vi "Manage Waypoint Shape.vi"(5 "Draw Arrow":bool, 6 "Coords":cluster{"x":dbl, "y":dbl}, 7 "Drawing Options":T1, 8 "Operation":enum16{"Draw", "Pt Test"}(ring), 9 "new picture in":picture, 10 "Waypoint Position (ft)":cluster{"x":dbl, "y":dbl, "th":dbl}, 11 "Pict Ref":refnum<vi>) -> (0 "Pt Test Results":enum16{"Miss", "Rect Hit", "Arrow Hit"}(ring), 1 "new picture out":picture)   [LabVIEW 2019]
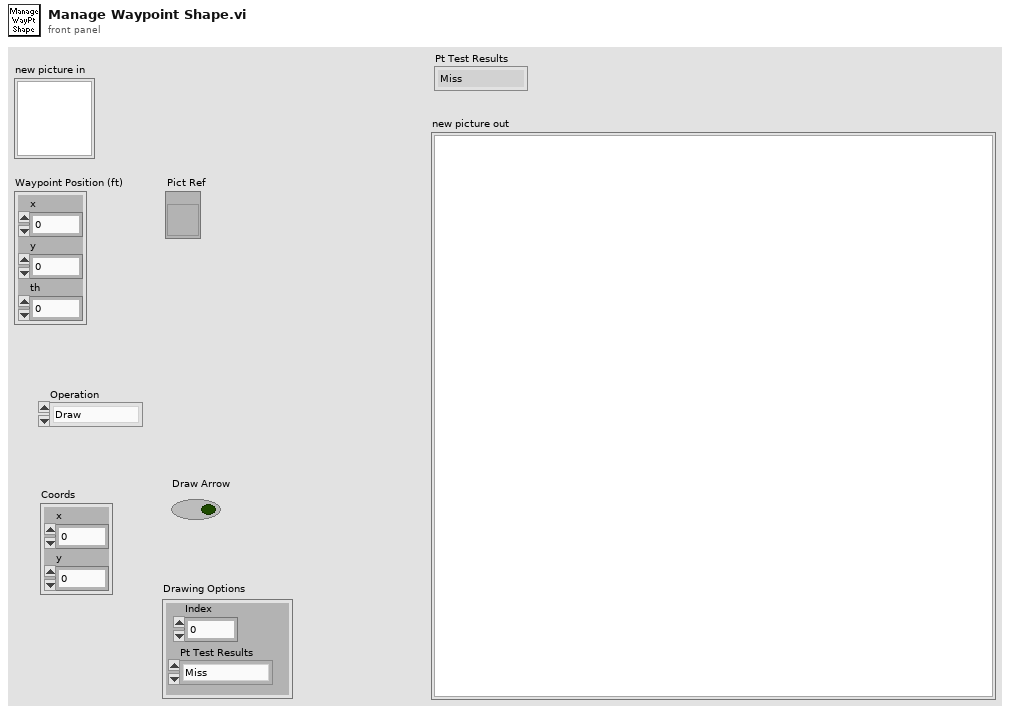
[diagram p1: front panel]
types:
  T1 = cluster{"Index":u32, "Pt Test Results":enum16{"Miss", "Rect Hit", "Arrow Hit"}}
  T2 = typedef "LVPositionTypeDef.ctl" = cluster{"Left":i32, "Top":i32}
  T3 = typedef "LVBoundsTypeDef.ctl" = cluster{"Width":u32, "Height":u32}
  T4 = cluster{"horizontal":enum16{"left", "center", "right"}, "vertical":enum16{"top", "center", "bottom"}}
  T5 = cluster{"Width":u16, "Style":enum32{"Solid", "Dash", "Dot", "DashDot", "DashDotDot"}}
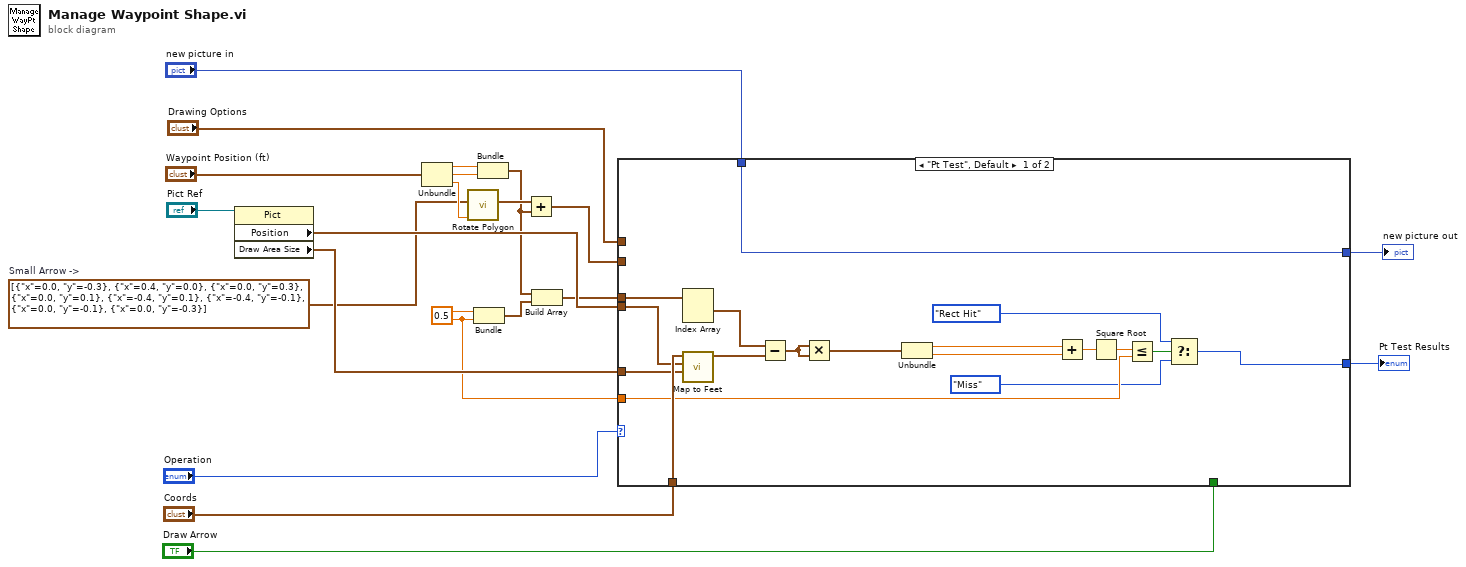
[diagram p0: block diagram]
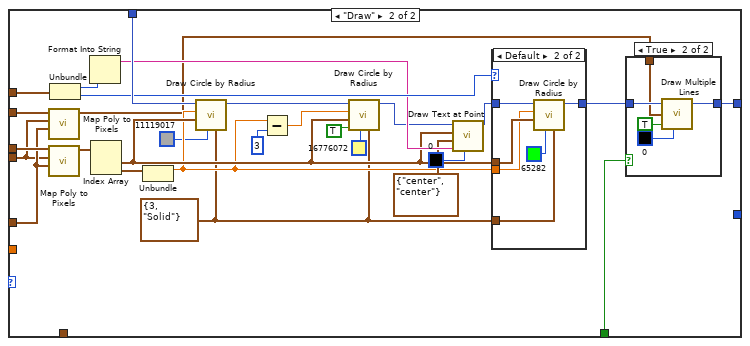
[diagram p2: hidden frame]
diagram:
  w5 = cluster{"x":dbl, "y":dbl}[] [{"x"=0.0, "y"=-0.3}, {"x"=0.4, "y"=0.0}, {"x"=0.0, "y"=0.3}, {"x"=0.0, "y"=0.1}, {"x"=-0.4, "y"=0.1}, {"x"=-0.4, "y"=-0.1}, {"x"=0.0, "y"=-0.1}, {"x"=0.0, "y"=-0.3}]  # Small Arrow ->
  w7 = 0.5 ("y")
  n1 = property on="Property Node" class="Pict"(reference="Pict Ref") -> ("Position"=w16:T2, "Draw Area Size"=w15:T3)  [unwired: 1 in, 2 out]
  n2 = Unbundle("Waypoint Position (ft)") -> ("x"=w18:dbl, "y"=w19:dbl, "th"=w6:dbl)
  n3 = call "Rotate Polygon.vi"("Angle"=w6, "polygon 2"=w5) -> ("polygon"=w4:cluster{dbl, dbl}[])  [unwired: 9 in]
  n4 = Bundle("y"=w7, "y"=w7) -> (w8:cluster{"y":dbl, "y":dbl})  [unwired: 1 in]
  n5 = Bundle("x"=w18, "y"=w19) -> (w3:cluster{"x":dbl, "y":dbl})  [unwired: 1 in]
  n6 = Add(x=w4, y=w3) -> (x+y=w2:cluster{dbl, dbl}[])
  n7 = Build Array(w3, w8) -> (w9:cluster{"y":dbl, "y":dbl}[])
  n8 = case shown="\"Pt Test\", Default" "Operation" {
    tunnel: w9 -> [w34 w65]
    tunnel: [w39 w45] -> w21
    tunnel: "new picture in" -> [w39 w66]
    tunnel: w16 -> [w36 w47]
    tunnel: w15 -> [w37 w48]
    tunnel: "Coords" -> [w38 _]
    tunnel: [w22 _] -> w11
    tunnel: "Drawing Options" -> [_ w67]
    tunnel: w7 -> [w26 _]
    tunnel: w2 -> [_ w49]
    tunnel: "Draw Arrow" -> [_ w43]
    frame "Pt Test", Default {
      n9 = Index Array(array=w34) -> (element #1=w33:cluster{"y":dbl, "y":dbl})  [unwired: 2 in, 1 out]
      n10 = call "Map to Feet.vi"("Draw Area Size"=w37, "Position"=w36, "Coords (px)"=w38) -> ("Point (ft)"=w35:cluster{dbl, dbl})  [unwired: 8 in]
      n11 = Subtract(x=w33, y=w35) -> (x-y=w32:cluster{dbl, dbl})
      n12 = Multiply(x=w32, y=w32) -> (x*y=w31:cluster{dbl, dbl})
      n13 = Unbundle(w31) -> (w30:dbl, w29:dbl)
      n14 = Add(x=w30, y=w29) -> (x+y=w28:dbl)
      n15 = Square Root(x=w28) -> (sqrt(x)=w27:dbl)
      n16 = Less Or Equal?(x=w27, y=w26) -> (x <= y?=w25:bool)
      n17 = Select(t=enum16{"Miss", "Rect Hit", "Arrow Hit"}."Rect Hit" ("Pt Test Results"), s=w25, f=enum16{"Miss", "Rect Hit", "Arrow Hit"}."Miss" ("Pt Test Results")) -> (s? t:f=w22:enum16{"Miss", "Rect Hit", "Arrow Hit"})
    }
    frame "Draw" {
      w42 = T5 {"Width"=3, "Style"=enum."Solid"} ("pen")
      n18 = call "Map Poly to Pixels.vi"("Draw Area Size"=w48, "Position"=w47, "Coords"=w49) -> ("Coords"=w44:cluster{"Horizontal":dbl, "Vertical":dbl}[])  [unwired: 8 in]
      n19 = call "Map Poly to Pixels.vi"("Draw Area Size"=w48, "Position"=w47, "Coords"=w65) -> ("Coords"=w64:cluster{"Horizontal":dbl, "Vertical":dbl}[])  [unwired: 8 in]
      n20 = Unbundle(w67) -> ("Index"=w61:u32, "Pt Test Results"=w62:enum16{"Miss", "Rect Hit", "Arrow Hit"})
      n21 = Format Into String(w61) -> (resulting string=w59:string)  [unwired: 3 in, 1 out]
      n22 = Index Array(array=w64) -> (element #1=w53:cluster{"Horizontal":dbl, "Vertical":dbl}, element #2=w63:cluster{"Horizontal":dbl, "Vertical":dbl})  [unwired: 2 in]
      n23 = Unbundle(w63) -> ("Horizontal"=w52:dbl)  [unwired: 1 out]
      n24 = call <vilib>:"Draw Circle by Radius.vi"("pen"=w42, "color(black)"=u32 11119017, "pixel center"=w53, "radius"=w52, "picture"=w66) -> ("new picture"=w57:picture)  [unwired: 6 in]
      n25 = Subtract(x=w52, y=u16 3 ("Width")) -> (x-y=w51:dbl)
      n26 = call <vilib>:"Draw Circle by Radius.vi"("pen"=w42, "color(black)"=u32 16776072, "fill?(F)"=TRUE, "pixel center"=w53, "radius"=w51, "picture"=w57) -> ("new picture"=w56:picture)  [unwired: 5 in]
      n27 = call <vilib>:"Draw Text at Point.vi"("text color(black)"=u32 0, "text"=w59, "alignment(left, top)"=T4 {"horizontal"=enum."center", "vertical"=enum."center"}, "origin"=w53, "picture"=w56) -> ("new picture"=w60:picture)  [unwired: 5 in, 1 out]
      n28 = case shown="Default" w62 {
        tunnel: w60 -> [w74 w80]
        tunnel: [w74 w79] -> w46
        tunnel: w53 -> [_ w78]
        tunnel: w52 -> [_ w77]
        tunnel: w42 -> [_ w75]
        frame "Miss" {
        }
        frame Default {
          n29 = call <vilib>:"Draw Circle by Radius.vi"("pen"=w75, "color(black)"=u32 65282, "pixel center"=w78, "radius"=w77, "picture"=w80) -> ("new picture"=w79:picture)  [unwired: 6 in]
        }
      }
      n30 = case shown="True" w43 {
        tunnel: w46 -> [w68 w73]
        tunnel: [w68 w72] -> w45
        tunnel: w44 -> [_ w71]
        frame False {
        }
        frame True {
          n31 = call <vilib>:"Draw Multiple Lines.vi"("picture"=w73, "line endpoints"=w71, "fill?(F)"=TRUE, "color(black)"=u32 0) -> ("new picture"=w72:picture)  [unwired: 5 in]
        }
      }
    }
  }
  "new picture out" <- w21
  "Pt Test Results" <- w11
